vi "Weight Motion.vi"(7 "Console Log in":refnum<class "Console Log.lvclass">, 8 "error in":errorcluster, 11 "Gluing Procedure in":refnum<class "Gluing Procedure.lvclass">) -> (0 "error out":errorcluster, 1 "Step canceled?":bool, 3 "Gluing Procedure out":refnum<class "Gluing Procedure.lvclass">, 5 "Console Log out":refnum<class "Console Log.lvclass">)   [LabVIEW 2011, in "Gluing Procedure.lvclass"]
uses:
  Gluing Procedure.lvclass
  Application Utilities/Console Log/Console Log.lvclass
  Type Definitions/Weight Placement.ctl
  Shared Components/GrabberTool Class/GrabberTool Class.lvclass
panel:
  # "This VI does the Weight motion.\n\n1.  grabber\n2.  grab weight\n3.  place weight\n4.  unload grabber\n\nneed weight -> bbm path motion (chuck/slot)"
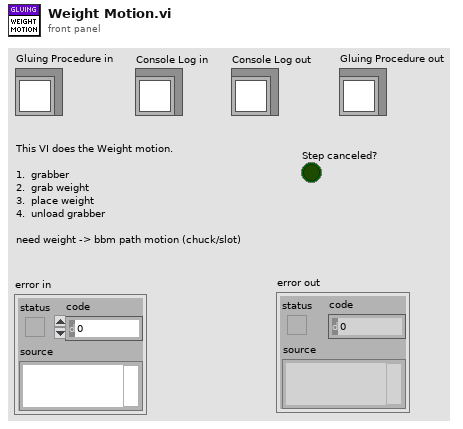
[diagram p1: front panel]
types:
  T1 = typedef "Weight Placement.ctl" = cluster{"Has been run?":bool}
  T2 = typedef "Configure.ctl" = cluster{"Has been run?":bool, "Active Paths":T3, "Glue Pathways":T4, "Chuck Module Used for BBM:":T6}
  T3 = typedef "Active Paths.ctl" = bool[]
  T4 = typedef "Glue Paths.ctl" = T5[]
  T5 = typedef "Glue Path.ctl" = cluster{"HDI Slot ":i32, "Stamp Slot":i32, "Glue Slot":i32, "Weight Slot":i32, "BBM Slot":i32}
  T6 = typedef "BBM Chuck Used.ctl" = i32
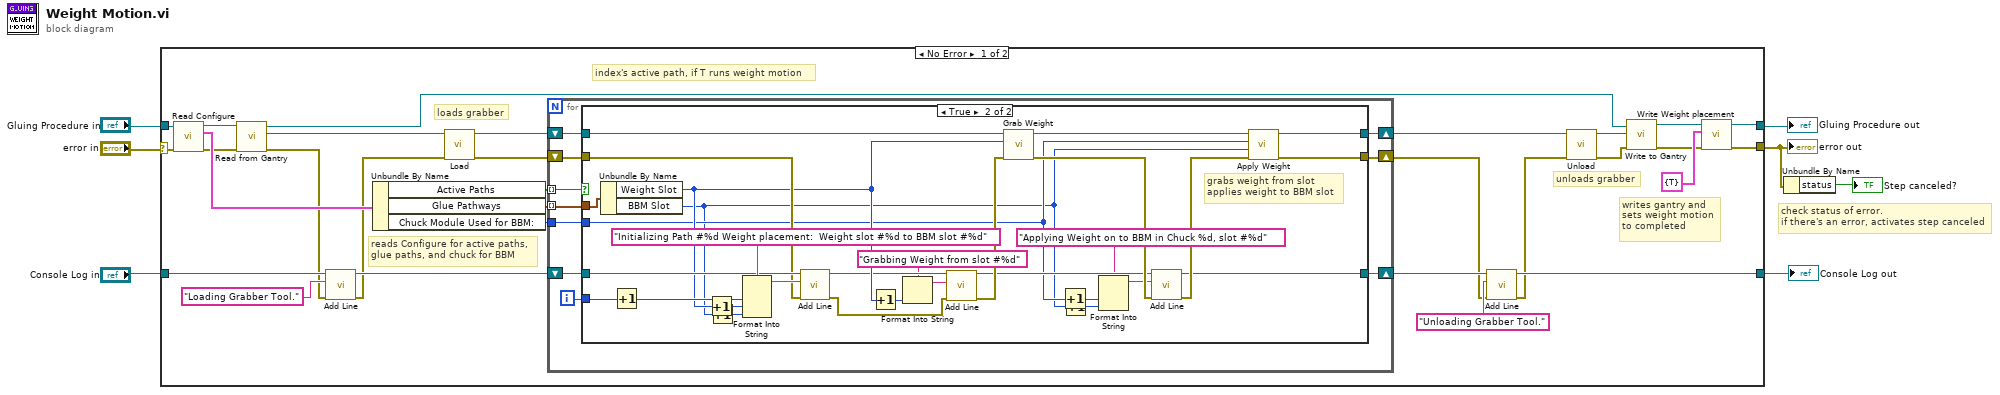
[diagram p0: block diagram]
diagram:
  # "check status of error.\nif there's an error, activates step canceled"
  n1 = case shown="No Error" "error in" {
    selector: "error in" -> [w36 w83]
    tunnel: [w18 w83] -> w3
    tunnel: [w19 w82] -> w5
    tunnel: "Gluing Procedure in" -> [w37 w82]
    tunnel: "Console Log in" -> [w17 w81]
    tunnel: [w10 w81] -> w1
    frame No Error {
      # "index's active path, if T runs weight motion"
      # "writes gantry and\nsets weight motion\nto completed"
      # "unloads grabber"
      # "reads Configure for active paths,\nglue paths, and chuck for BBM"
      # "loads grabber"
      n2 = call "Read Configure.vi"("error in (no error)"=w36, "Gluing Procedure in"=w37) -> ("error out"=w33:errorcluster, "Configure"=w34:T2, "Gluing Procedure out"=w35:refnum<class "Gluing Procedure.lvclass">)  [unwired: 7 in]
      n3 = call "Read from Gantry.vi"("error in (no error)"=w33, "Gluing Procedure in"=w35) -> ("error out"=w14:errorcluster, "Gantry"=w32:refnum<class "Gantry Class.lvclass">, "Gluing Procedure out"=w25:refnum<class "Gluing Procedure.lvclass">)  [unwired: 7 in]
      n4 = call "Add Line.vi"("error in"=w14, "String"="Loading Grabber Tool.", "Console Log in"=w17) -> ("error out"=w13:errorcluster, "Console Log out"=w15:refnum<class "Console Log.lvclass">)  [unwired: 7 in]
      n5 = Unbundle By Name(w34) -> ("Active Paths"=w31:T3, "Glue Pathways"=w30:T4, "Chuck Module Used for BBM:"=w29:T6)
      n6 = call "Load.vi"("error in"=w13, "Gantry In"=w32) -> ("error out"=w27:errorcluster, "Grabber Tool out"=w28:refnum<class "GrabberTool Class.lvclass">)  [unwired: 8 in]
      n7 = for {
        tunnel: w31 -> [w47] mode=indexing
        tunnel: w30 -> [w44] mode=indexing
        tunnel: w29 -> [w43]
        shift-right: [w42] -> w26
        shift-left: w28 -> [w46]
        shift-right: [w41] -> w9
        shift-left: w27 -> [w45]
        shift-right: [w39] -> w12
        shift-left: w15 -> [w38]
        i -> [w40]
        n8 = case shown="True" w47 {
          tunnel: w46 -> [w50 w79]
          tunnel: w45 -> [w49 w68]
          tunnel: w44 -> [_ w80]
          tunnel: w43 -> [_ w55]
          tunnel: [w50 w77] -> w42
          tunnel: [w49 w76] -> w41
          tunnel: w40 -> [_ w75]
          tunnel: w38 -> [w48 w71]
          tunnel: [w48 w51] -> w39
          frame False {
          }
          frame True {
            # "grabs weight from slot\napplies weight to BBM slot"
            n9 = Unbundle By Name(w80) -> ("Weight Slot"=w65:i32, "BBM Slot"=w54:i32)
            n10 = Increment(x=w75) -> (x+1=w74:i32)
            n11 = Increment(x=w65) -> (x+1=w70:i32)
            n12 = Increment(x=w54) -> (x+1=w69:i32)
            n13 = Format Into String(format string="Initializing Path #%d Weight placement:  Weight slot #%d to BBM slot #%d", w74, w70, w69) -> (resulting string=w72:string)  [unwired: 2 in, 1 out]
            n14 = call "Add Line.vi"("error in"=w68, "String"=w72, "Console Log in"=w71) -> ("error out"=w60:errorcluster, "Console Log out"=w64:refnum<class "Console Log.lvclass">)  [unwired: 7 in]
            n15 = Increment(x=w65) -> (x+1=w67:i32)
            n16 = Format Into String(format string="Grabbing Weight from slot #%d", w67) -> (resulting string=w66:string)  [unwired: 2 in, 1 out]
            n17 = call "Add Line.vi"("error in"=w60, "String"=w66, "Console Log in"=w64) -> ("error out"=w62:errorcluster, "Console Log out"=w58:refnum<class "Console Log.lvclass">)  [unwired: 7 in]
            n18 = call "Grab Weight.vi"("error in"=w62, "Weight Number"=w65, "GrabberTool in"=w79) -> ("error out"=w61:errorcluster, "GrabberTool out"=w78:refnum<class "GrabberTool Class.lvclass">)  [unwired: 7 in]
            n19 = Increment(x=w55) -> (x+1=w57:T6)
            n20 = Increment(x=w54) -> (x+1=w56:i32)
            n21 = Format Into String(format string="Applying Weight on to BBM in Chuck %d, slot #%d", w57, w56) -> (resulting string=w59:string)  [unwired: 2 in, 1 out]
            n22 = call "Add Line.vi"("error in"=w61, "String"=w59, "Console Log in"=w58) -> ("error out"=w52:errorcluster, "Console Log out"=w51:refnum<class "Console Log.lvclass">)  [unwired: 7 in]
            n23 = call "Apply Weight.vi"("error in"=w52, "Slot Number"=w54, "Chuck Number"=w55, "GrabberTool in"=w78) -> ("error out"=w76:errorcluster, "GrabberTool out"=w77:refnum<class "GrabberTool Class.lvclass">)  [unwired: 6 in]
          }
        }
      }
      n24 = call "Add Line.vi"("error in"=w9, "String"="Unloading Grabber Tool.", "Console Log in"=w12) -> ("error out"=w8:errorcluster, "Console Log out"=w10:refnum<class "Console Log.lvclass">)  [unwired: 7 in]
      n25 = call "Unload.vi"("error in"=w8, "GrabberTool in"=w26) -> ("error out"=w23:errorcluster, "Gantry out"=w24:refnum<class "Gantry Class.lvclass">)  [unwired: 8 in]
      n26 = call "Write to Gantry.vi"("error in (no error)"=w23, "Gantry"=w24, "Gluing Procedure in"=w25) -> ("error out"=w20:errorcluster, "Gluing Procedure out"=w22:refnum<class "Gluing Procedure.lvclass">)  [unwired: 7 in]
      n27 = call "Write Weight placement.vi"("error in (no error)"=w20, "Weight placement"=T1 {"Has been run?"=TRUE}, "Gluing Procedure in"=w22) -> ("error out"=w18:errorcluster, "Gluing Procedure out"=w19:refnum<class "Gluing Procedure.lvclass">)  [unwired: 7 in]
    }
    frame Error {
    }
  }
  "error out" <- w3
  "Gluing Procedure out" <- w5
  "Console Log out" <- w1
  n28 = Unbundle By Name(w3) -> ("status"=→"Step canceled?":bool)
